vi "GetActualShoulderAngleData.vi"(11 "Reset Encoder":bool) -> (2 "Encoder Speed (deg/s)":dbl, 3 "Encoder Angle (deg)":dbl)   [LabVIEW 2018]
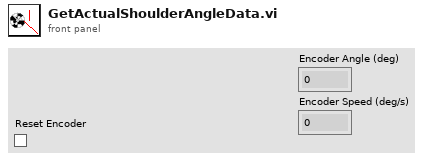
[diagram p1: front panel]
types:
  T1 = typedef "WPI_EncoderDevRef.ctl" = cluster{"DevStatus":errorcluster, "EncoderIndex":T2, "CounterIndex":T3, "DistancePerCount":dbl, "Decoding Type":T4}
  T2 = typedef "FPGA_EncoderIdx.ctl" = enum8{"Enc 0", "Enc 1", "Enc 2", "Enc 3", "Enc 4", "Enc 5", "Enc 6", "Enc 7", "Invalid"}
  T3 = typedef "FPGA_CounterCtrSystemIndex.ctl" = enum8{"Ctr 0", "Ctr 1", "Ctr 2", "Ctr 3", "Ctr 4", "Ctr 5", "Ctr 6", "Ctr 7", "Invalid"}
  T4 = typedef "WPI_EncoderType.ctl" = enum16{"1x", "2x", "4x"}
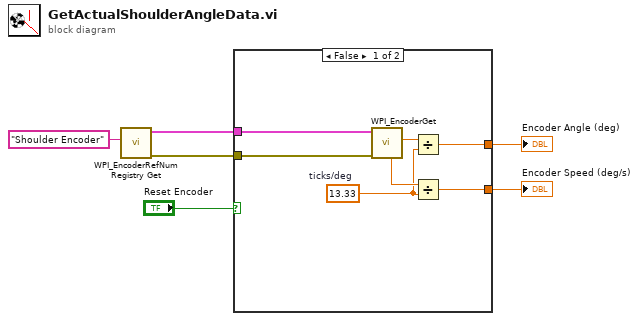
[diagram p0: block diagram]
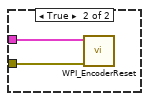
[diagram p2: hidden frame]
diagram:
  n1 = call <vilib>:"WPI_EncoderRefNum Registry Get.vi"("refnum name"="Shoulder Encoder") -> ("error out"=w4:errorcluster, "EncoderDevRef"=w6:T1)  [unwired: 9 in]
  n2 = case shown="False" "Reset Encoder" {
    tunnel: w6 -> [w13 w15]
    tunnel: w4 -> [w12 w14]
    tunnel: [w8 _] -> w3
    tunnel: [w7 _] -> w2
    frame False {
      w9 = 13.33  # ticks/deg
      n3 = call <vilib>:"WPI_EncoderGet.vi"("error in (no error)"=w12, "EncoderDevRef"=w13) -> ("Distance"=w11:dbl, "Rate"=w10:dbl)  [unwired: 4 in, 4 out]
      n4 = Divide(x=w11, y=w9) -> (x/y=w8:dbl)
      n5 = Divide(x=w10, y=w9) -> (x/y=w7:dbl)
    }
    frame True {
      n6 = call <vilib>:"WPI_EncoderReset.vi"("error in (no error)"=w14, "EncoderDevRef"=w15) -> ()  [unwired: 8 in, 2 out]
    }
  }
  "Encoder Angle (deg)" <- w3
  "Encoder Speed (deg/s)" <- w2
